vi "例10.10  读取avi文件.vi"() -> ()   [LabVIEW 2017]
panel:
  in  "stop":bool
  out "Image":T1(plugin-control)
  out "Start Time":u32
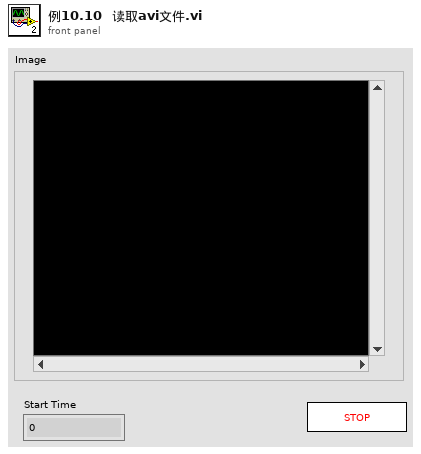
[diagram p1: front panel]
types:
  T1 = typedef "IMAQ Image.ctl" = refnum<image>
  T2 = typedef "AviRefnum.ctl" = refnum<k1>
  T3 = typedef "Image Type" = u32
  T4 = cluster{"width":u32, "height":u32, "framesPerSecond":u32, "compressionFilter":string, "hasData":bool}
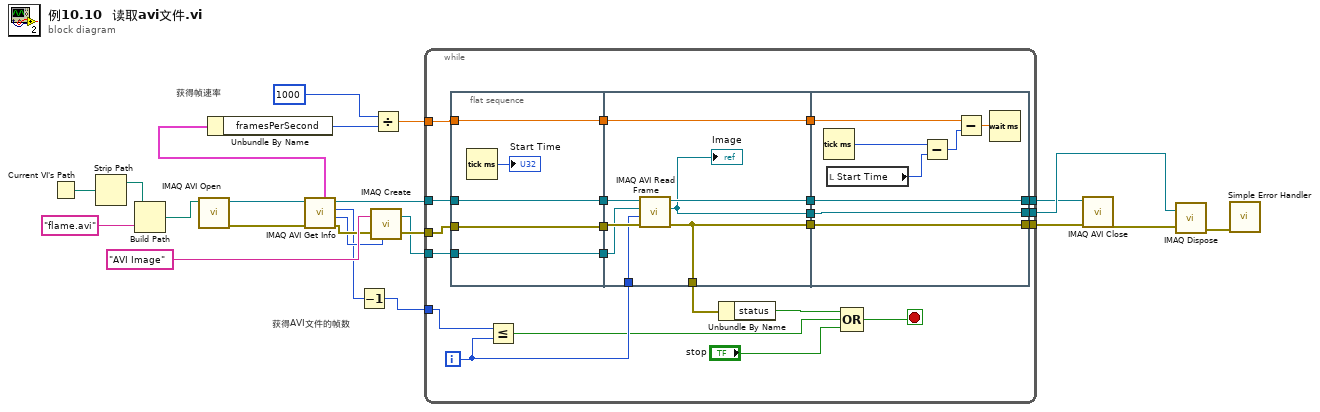
[diagram p0: block diagram]
diagram:
  # "获得帧速率"
  # "获得AVI文件的帧数"
  n1 = Current VI's Path ("当前VI路径")() -> (path=w1:path)
  n2 = Strip Path ("拆分路径")(path=w1) -> (stripped path=w5:path)  [unwired: 1 out]
  n3 = Build Path ("创建路径")(base path=w5, name or relative path="flame.avi") -> (appended path=w4:path)
  n4 = call "IMAQ AVI Open"("AVI Path"=w4) -> ("error out"=w17:errorcluster, "Avi Refnum"=w16:T2)  [unwired: 1 in, 8 out]
  n5 = call "IMAQ AVI Get Info"("error in (no error)"=w17, "Avi Refnum"=w16) -> ("error out"=w14:errorcluster, "Image Type"=w8:T3, "Number of Frames"=w7:u32, "Avi Refnum (duplicate)"=w2:T2, "Frame Data"=w21:T4)  [unwired: 5 out]
  n6 = Unbundle By Name(w21) -> ("framesPerSecond"=w18:u32)
  n7 = Decrement(x=w7) -> (x-1=w9:u32)
  n8 = call "IMAQ Create"("Image Name"="AVI Image", "Image Type"=w8, "error in (no error)"=w14) -> ("New Image"=w12:T1, "error out"=w13:errorcluster)  [unwired: 1 in, 1 out]
  n9 = Divide(x=1000, y=w18) -> (x/y=w19:dbl)
  n10 = while {
    tunnel: w12 -> [w41]
    tunnel: [w43] -> w3
    tunnel: [w27] -> w15
    tunnel: w19 -> [w40]
    tunnel: w13 -> [w44]
    tunnel: w2 -> [w45]
    tunnel: [w30] -> w10
    tunnel: w9 -> [w39]
    i -> [w29]
    stop <- w42 stop-if-true
    n11 = flat-sequence {
      tunnel: w45 -> [w49]
      tunnel: [w49] -> w38
      tunnel: w44 -> [w48]
      tunnel: [w48] -> w37
      tunnel: w41 -> [w47]
      tunnel: [w47] -> w36
      tunnel: w40 -> [w46]
      tunnel: [w46] -> w35
      tunnel: w38 -> [w58]
      tunnel: w37 -> [w57]
      tunnel: [w56] -> w34
      tunnel: w36 -> [w55]
      tunnel: [w53] -> w33
      tunnel: w35 -> [w54]
      tunnel: [w54] -> w32
      tunnel: [w51] -> w31
      tunnel: w29 -> [w52]
      tunnel: [w51] -> w26
      tunnel: [w62] -> w43
      tunnel: w34 -> [w62]
      tunnel: [w59] -> w30
      tunnel: w33 -> [w59]
      tunnel: w32 -> [w63]
      tunnel: [w61] -> w27
      tunnel: w31 -> [w61]
      frame #0 {
        n12 = Tick Count (ms)() -> (millisecond timer value=→"Start Time":u32)
      }
      frame #1 {
        n13 = call "IMAQ AVI Read Frame"("error in (no error)"=w57, "Frame Number"=w52, "Image"=w55, "Avi Refnum"=w58) -> ("error out"=w51:errorcluster, "Image Out"=w53:T1, "Avi Refnum (duplicate)"=w56:T2)  [unwired: 1 in, 4 out]
        "Image" <- w53
      }
      frame #2 {
        n14 = Tick Count (ms)() -> (millisecond timer value=w66:u32)
        n15 = local read "Start Time"() -> (w65:u32)
        n16 = Subtract(x=w66, y=w65) -> (x-y=w64:u32)
        n17 = Subtract(x=w63, y=w64) -> (x-y=w60:dbl)
        n18 = Wait (ms)(milliseconds to wait=w60) -> ()  [unwired: 1 out]
      }
    }
    n19 = Less Or Equal?(x=w39, y=w29) -> (x <= y?=w24:bool)
    n20 = Unbundle By Name(w26) -> ("status"=w25:bool)
    n21 = Compound Arithmetic op=OR(w25, w24, "stop") -> (w42:bool)
  }
  n22 = call "IMAQ AVI Close"("error in (no error)"=w15, "Avi Refnum"=w3) -> ("error out"=w11:errorcluster)  [unwired: 9 out]
  n23 = call "IMAQ Dispose"("Image"=w10, "error in (no error)"=w11) -> ("error out"=w22:errorcluster)  [unwired: 1 in, 3 out]
  n24 = call <vilib>:"Simple Error Handler.vi"("error in (no error)"=w22) -> ()  [unwired: 1 in, 8 out]
